vi "Mono (YJ) - JPJ.vi"(3 "error in (no error)":errorcluster, 5 "Go to Wavelength":dbl, 6 "CmdLib In":refnum<k24>) -> (0 "error out 2":errorcluster, 1 "State of Mono_SetWavelength":bool=TRUE, 2 "Current Wavelength":dbl)   [LabVIEW 2023]
uses:
  E:/Old PC/desktop/Sensitive EQE Stuff/S-EQE (YJ)/Mono vi (YJ)/Cornerstone.dll
  Cornerstone.dll
panel:
  out "Numeric":i32
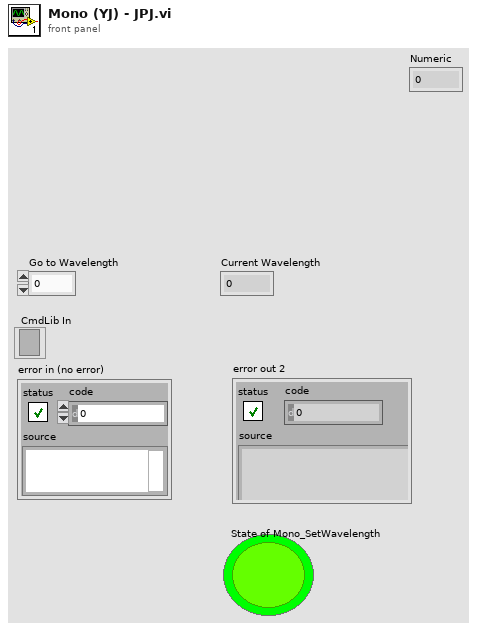
[diagram p1: front panel]
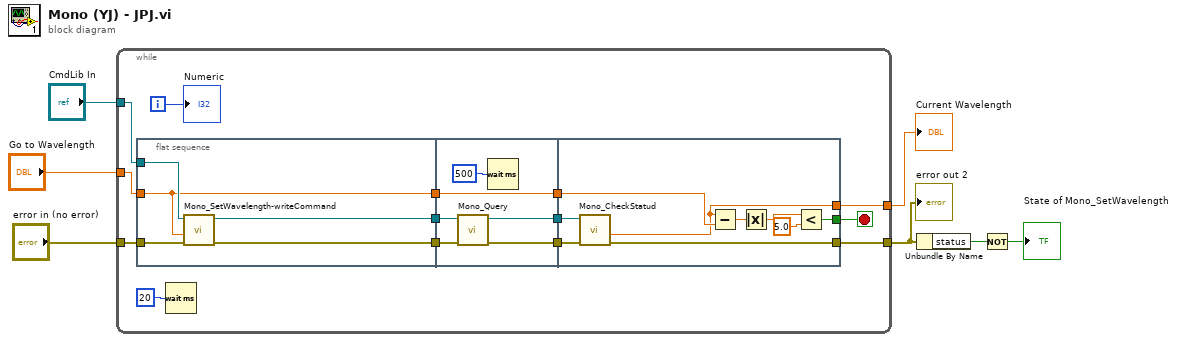
[diagram p0: block diagram]
diagram:
  n1 = while {
    tunnel: "error in (no error)" -> [w19]
    tunnel: "CmdLib In" -> [w18]
    tunnel: [w17] -> w5
    tunnel: [w16] -> w2
    tunnel: "Go to Wavelength" -> [w15]
    i -> [w14]
    stop <- w21 stop-if-true
    n2 = flat-sequence {
      tunnel: [w25] -> w13
      tunnel: [w24] -> w11
      tunnel: [w22] -> w10
      tunnel: w19 -> [w26]
      tunnel: w18 -> [w23]
      tunnel: w15 -> [w22]
      tunnel: w13 -> [w30]
      tunnel: [w29] -> w12
      tunnel: w11 -> [w31]
      tunnel: w10 -> [w32]
      tunnel: [w32] -> w9
      tunnel: [w28] -> w8
      tunnel: w12 -> [w40]
      tunnel: w9 -> [w39]
      tunnel: [w35] -> w21
      tunnel: [w34] -> w17
      tunnel: [w33] -> w16
      tunnel: w8 -> [w41]
      frame #0 {
        n3 = call "Mono_SetWavelength-writeCommand.vi"("error in (no error) 2"=w26, "Wavelength"=w22, "CmdLib In"=w23) -> ("error out 2"=w25:errorcluster, "CmdLib Out"=w24:refnum<k24>)  [unwired: 6 in, 1 out]
      }
      frame #1 {
        n4 = call "Mono_Query.vi"("error in (no error) 2"=w30, "CmdLib In"=w31) -> ("error out 2"=w29:errorcluster, "CmdLib Out"=w28:refnum<k24>)  [unwired: 8 in]
        n5 = Wait (ms)(milliseconds to wait=u32 500) -> ()  [unwired: 1 out]
      }
      frame #2 {
        n6 = call "Mono_CheckStatud.vi"("error in (no error) 2"=w40, "CmdLib In"=w41) -> ("error out 2"=w34:errorcluster, "getWavelength"=w33:dbl)  [unwired: 7 in, 1 out]
        n7 = Subtract(x=w33, y=w39) -> (x-y=w38:dbl)
        n8 = Absolute Value(x=w38) -> (abs(x)=w37:dbl)
        n9 = Less?(x=w37, y=5.0) -> (x < y?=w35:bool)
      }
    }
    n10 = Wait (ms)(milliseconds to wait=u32 20) -> ()  [unwired: 1 out]
    "Numeric" <- w14
  }
  "error out 2" <- w5
  "Current Wavelength" <- w2
  n11 = Unbundle By Name(w5) -> ("status"=w4:bool)
  n12 = Not(x=w4) -> (.not. x?=→"State of Mono_SetWavelength":bool)
